vi "invalid attribute names.vi"() -> ()   [LabVIEW 2019]
panel:
  out "Error Out":errorcluster
  in  "TDMS File":path=path "C:/Python/projects/nitdms/tests/tdms_files/invalid attributes names.tdms"
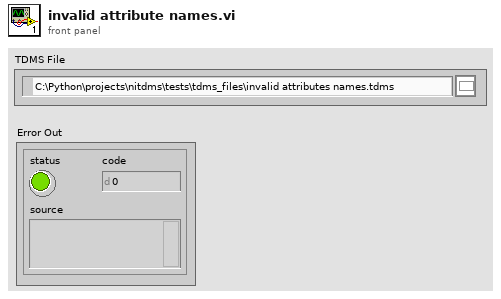
[diagram p1: front panel]
types:
  T1 = enum16{"open", "open or create", "create or replace", "create", "open (read-only)"}
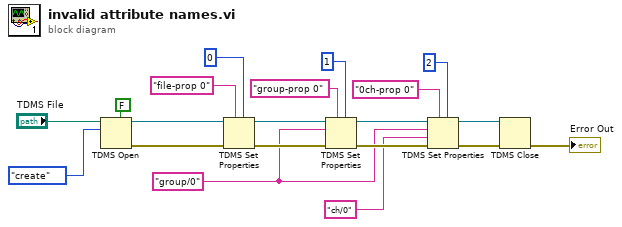
[diagram p0: block diagram]
diagram:
  w5 = "group/0"
  n1 = TDMS Open(5:FALSE ("create index file? (T)"), 10:T1."create" ("operation (0:open)"), 11:"TDMS File") -> (0:w16:errorcluster, 3:w15:refnum<k34>)  [unwired: 4 in]
  n2 = TDMS Set Properties(5:0, 7:"file-prop 0", 8:w16, 11:w15) -> (0:w12:errorcluster, 3:w11:refnum<k34>)  [unwired: 2 in, 2 out]
  n3 = TDMS Set Properties(5:1, 7:"group-prop 0", 8:w12, 10:w5, 11:w11) -> (0:w6:errorcluster, 3:w4:refnum<k34>)  [unwired: 1 in, 2 out]
  n4 = TDMS Set Properties(5:2, 7:"0ch-prop 0", 8:w6, 9:"ch/0", 10:w5, 11:w4) -> (0:w2:errorcluster, 3:w1:refnum<k34>)  [unwired: 2 out]
  n5 = TDMS Close(8:w2, 11:w1) -> (0:→"Error Out":errorcluster)  [unwired: 1 out]
